vi "GetPlotRanges.vi"(11 "plots":refnum<vi>[](array[refnum])) -> (2 "Yscales":T1[](array[typedef]), 3 "Xscales":T1[](array[typedef]))   [LabVIEW 2022 SP3]
uses:
  <vilib>/Utility/miscctls.llb/LVRangeTypeDef.ctl
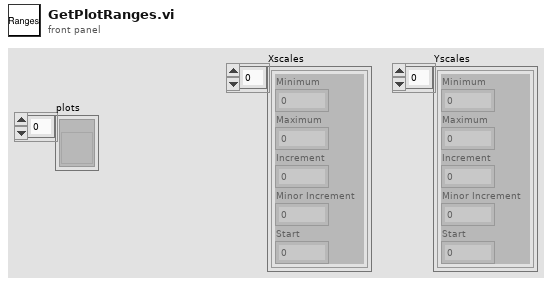
[diagram p1: front panel]
types:
  T1 = typedef "LVRangeTypeDef.ctl" = cluster{"Minimum":dbl, "Maximum":dbl, "Increment":dbl, "Minor Increment":dbl, "Start":dbl}
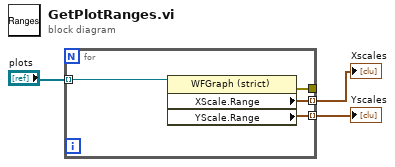
[diagram p0: block diagram]
diagram:
  n1 = for {
    tunnel: "plots" -> [w7] mode=indexing
    tunnel: [w6] -> w2 mode=indexing
    tunnel: [w5] -> w3 mode=indexing
    tunnel: [w4] -> _
    n2 = property class="WFGraph (strict)"(reference=w7) -> (error out=w4:errorcluster, "XScale.Range"=w6:T1, "YScale.Range"=w5:T1)  [unwired: 1 in, 1 out]
  }
  "Yscales" <- w3
  "Xscales" <- w2
